vi "MFC_Fault_Reset.vi"(8 "Previous Fault Array":bool[](array[boolean]), 10 "Reset":u8[](array[numeric])=[0, 0, 0, 0, 0, 0, 0, 0, 0, 0, 0, 0, 0, 0, 0, 0, 0, 0, 0, 0, 0, 0, 0, 0, 0], 11 "MFC Fault In Array":bool[](array[boolean])) -> (0 "Fault Out Array":bool[](array[boolean]))   [LabVIEW 2014]
panel:
  # "Output"
  # "Input"
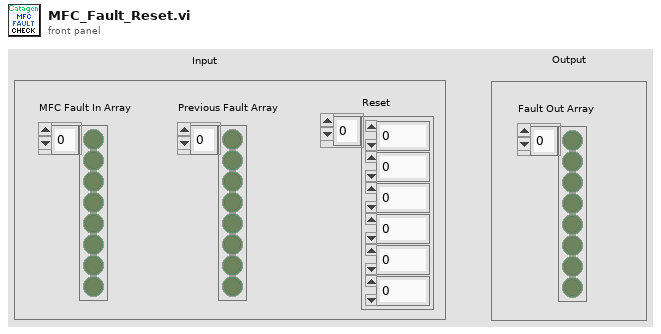
[diagram p1: front panel]
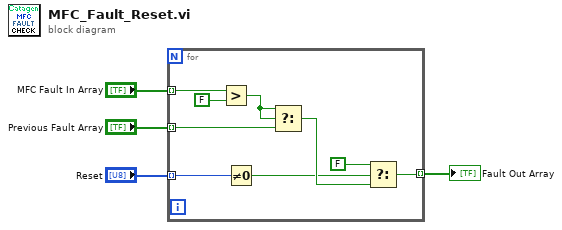
[diagram p0: block diagram]
diagram:
  n1 = for {
    tunnel: [w10] -> w4 mode=indexing
    tunnel: "MFC Fault In Array" -> [w9] mode=indexing
    tunnel: "Previous Fault Array" -> [w8] mode=indexing
    tunnel: "Reset" -> [w5] mode=indexing
    n2 = Greater?(x=w9, y=FALSE) -> (0:w11:bool)
    n3 = Not Equal To 0?(x=w5) -> (x != 0?=w6:bool)
    n4 = Select(t=w11, s=w11, f=w8) -> (s? t:f=w13:bool)
    n5 = Select(t=FALSE ("y"), s=w6, f=w13) -> (s? t:f=w10:bool)
  }
  "Fault Out Array" <- w4
